vi "ble_read_hr_monitor.vi"() -> ()   [LabVIEW 2013]
uses:
  type_def/connection_status_bundle.ctl
  type_def/address_type.ctl
panel:
  out "Reading HR":bool
  in  "stop":bool
  out "HR (bpm)":u16
  out "Connected":bool
  out "Device Name":string
  in  "Address Type":T1=1 items=["Public", "Random"]
  out "Handle table":string[][](array[string])
  out "Connection Status":T2={"MAC Address"="", "cnx handle"=0, "cnx flags"=0, "Address Type"=125, "Connection Interval (ms)"=125, "Timeout(ms)"=125, "Latency"=0, "bonding handle"=0} {"Address Type" items=["Public", "Random"]}
  out "Scanning":bool
  in  "Continue":bool
  in  "MAC Address":string
  in  "COM Bluegiga in":refnum<visa-resource-name>="COM13"
  out "Devices":string[][](array[string])
  out "BLED112 Dongle Info":string
  # "This VI an example of scanning for BLE devices using the \nBLED112 Bluetooth Smart Dongle by Bluegiga\nhttps://www.bluegiga.com/en-US/products/bled112-bluetooth-smart-dongle/\nand\nBLE  toolkit for LabVIEW\n\nInstructions:\nBefore running the VI\n1. Select the COM port for the BLED112 USB receiver\n(You can verify this in the Device Manager)\n\n2. Run the VI\n\n3. The VI will reset the dongle and scan for available BLE devices\n \n4. Introduce the MAC Address and Address Type of the HR monitor to connect and click in the CONTINUE button to connect with it\n\nYour device MUST compy with the BLE Heart Rate Profile\nhttps://developer.bluetooth.org/TechnologyOverview/Pages/HRP.aspx\n\n5. The VI will read the Characteristic 0x2A00 of the Service 0x1800 which contains \nthe Device Name\n\nhttps://www.bluetooth.com/specifications/gatt/viewer?attributeXmlFile=org.bluetooth.service.generic_access.xml&u=org.bluetooth.service.generic_access.xml\n\n6. Hear rate value will be updated\n\n7. Click in STOP to end the Hear Rate acqusition"
  # "SCAN"
  # "RSSI (power)"
  # "Advertising Package Type"
  # "MAC Address"
  # "Address Type"
  # "Friendly name"
  # "DEVICES FOUND"
  # "Introduce the MAC Address and Address Type of the device you want to connect and click in the CONTINUE button"
  # "CONNECT"
  # "READING DATA FROM DEVICE"
  # "Service 0x1800\nCharacteristic 0x2A00\nDevice Name"
  # "Service 0x180D\nCharacteristic 0x2A37\nHeart Rate Measurement"
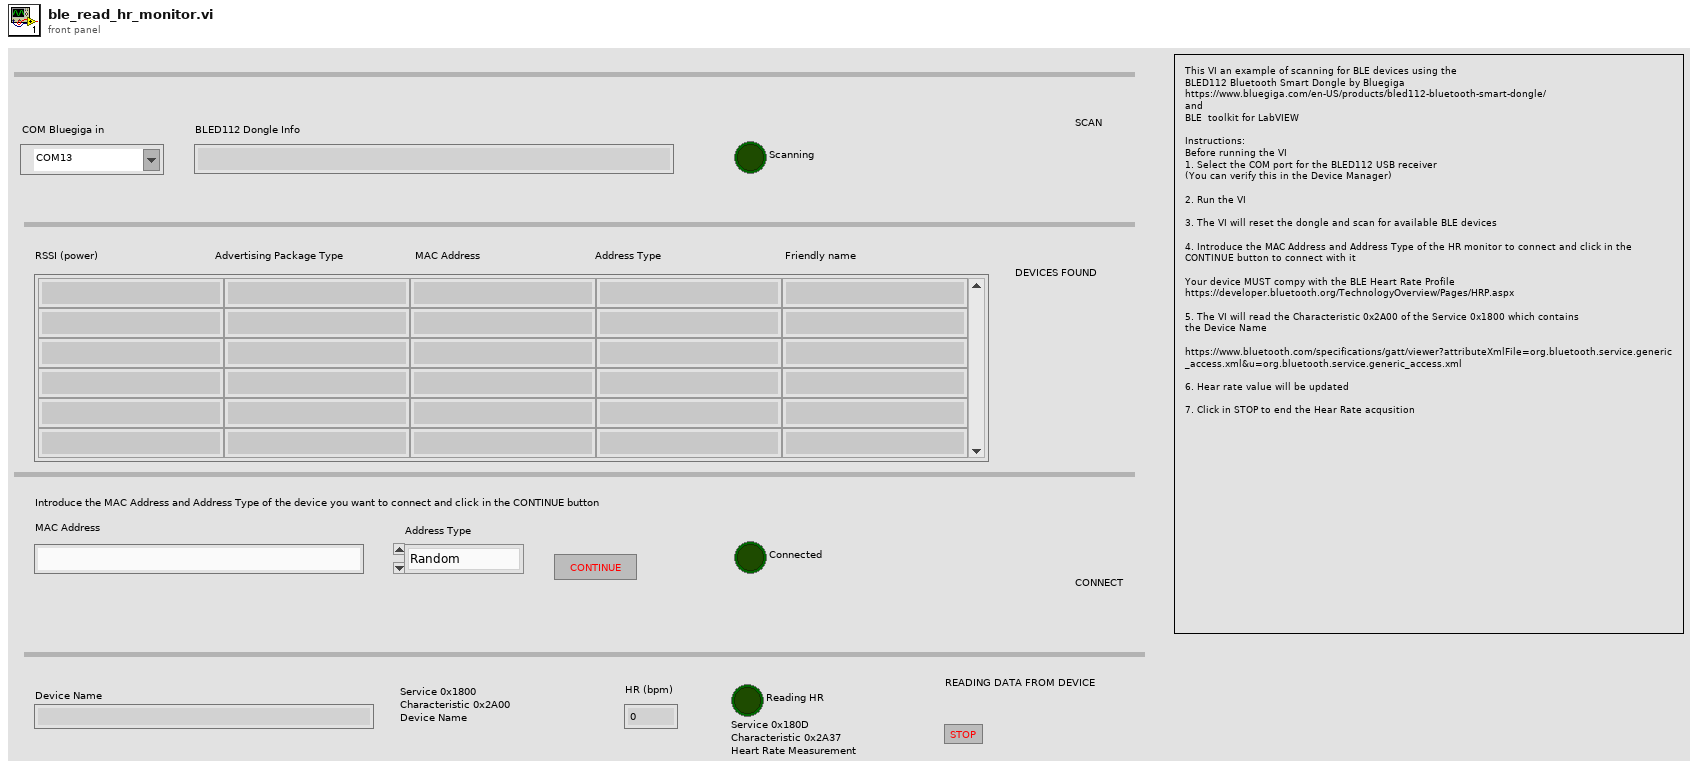
[diagram p1: front panel]
types:
  T1 = typedef "address_type.ctl" = u8
  T2 = typedef "connection_status_bundle.ctl" = cluster{"MAC Address":string, "cnx handle":u8, "cnx flags":u8, "Address Type":T1, "Connection Interval (ms)":u16, "Timeout(ms)":u16, "Latency":u16, "bonding handle":u8}
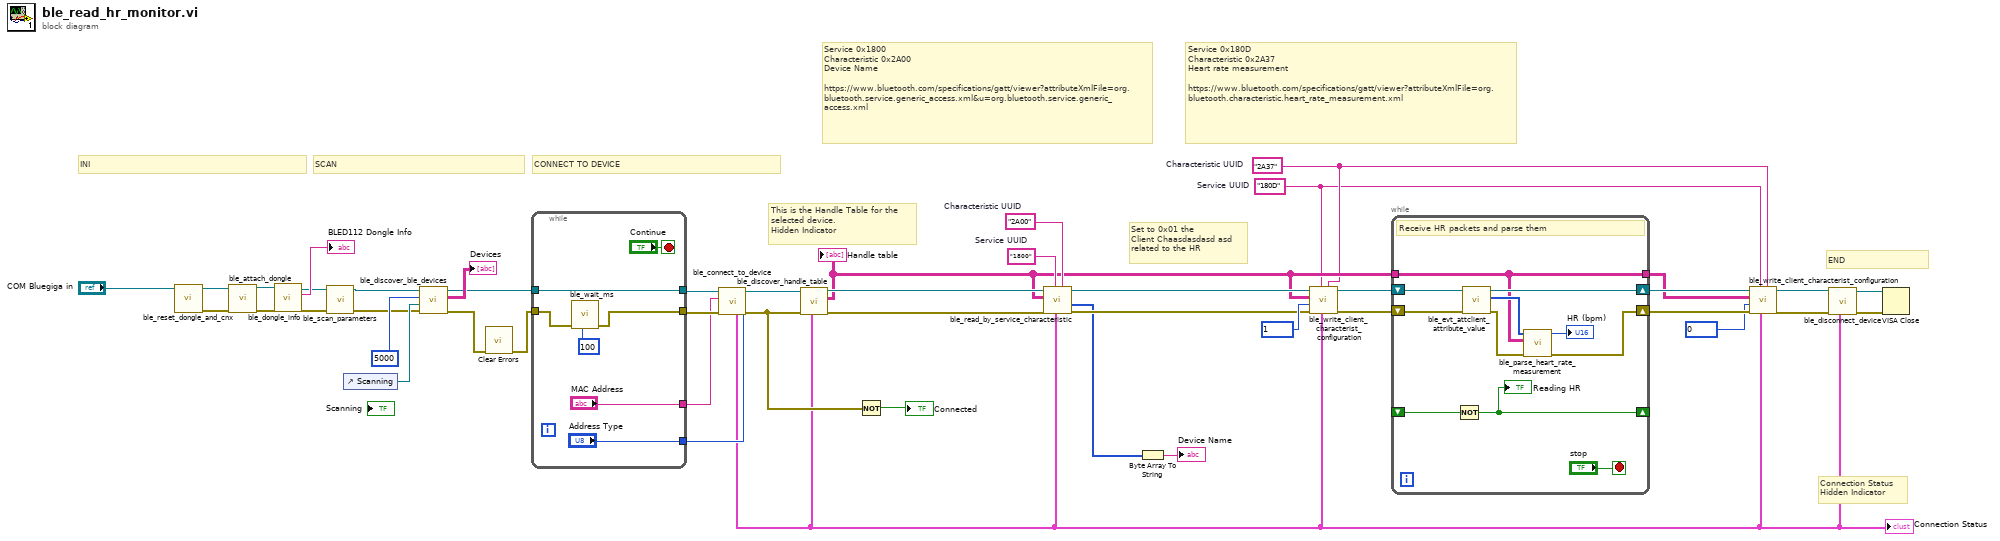
[diagram p0: block diagram]
diagram:
  w3 = "2A37"  # Characteristic UUID
  w2 = "180D"  # Service UUID
  w20 = "2A00"  # Characteristic UUID
  w21 = "1800"  # Service UUID
  # "Service 0x180D\nCharacteristic 0x2A37\nHeart rate measurement\n\nhttps://www.bluetooth.com/specifications/gatt/viewer?attributeXmlFile=org.bluetooth.characteristic.heart_rate_measurement.xml"
  # "Set to 0x01 the \nClient Chaasdasdasd asd\nrelated to the HR"
  # "Connection Status\nHidden Indicator"
  # "Service 0x1800\nCharacteristic 0x2A00\nDevice Name\n\nhttps://www.bluetooth.com/specifications/gatt/viewer?attributeXmlFile=org.bluetooth.service.generic_access.xml&u=org.bluetooth.service.generic_access.xml"
  # "This is the Handle Table for the\nselected device. \nHidden Indicator"
  # "CONNECT TO DEVICE"
  # "SCAN"
  # "END"
  # "INI"
  n1 = call "ble_reset_dongle_and_cnx.vi"("COM Bluegiga in"="COM Bluegiga in") -> ("error out"=w30:errorcluster, "COM Bluegiga out"=w28:refnum<visa-resource-name>)  [unwired: 9 in]
  n2 = call "ble_attach_dongle.vi"("error in (no error)"=w30, "COM Bluegiga in"=w28) -> ("error out"=w32:errorcluster, "COM Bluegiga out"=w31:refnum<visa-resource-name>)  [unwired: 8 in]
  n3 = call "ble_dongle_info.vi"("error in (no error)"=w32, "COM Bluegiga in"=w31) -> ("error out"=w38:errorcluster, "info"=→"BLED112 Dongle Info":string, "COM Bluegiga out"=w39:refnum<visa-resource-name>)  [unwired: 7 in]
  n4 = call "ble_scan_parameters.vi"("error in (no error)"=w38, "COM Bluegiga in"=w39) -> ("error out"=w36:errorcluster, "COM Bluegiga out"=w37:refnum<visa-resource-name>)  [unwired: 7 in, 1 out]
  n5 = control-ref of="Scanning"() -> (w42:refnum<vi>)
  n6 = call "ble_discover_ble_devices.vi"("error in (no error)"=w36, "LED ref"=w42, "Scan Duration (10000ms)"=u32 5000, "COM Bluegiga in"=w37) -> ("error out"=w26:errorcluster, "Devices"=→"Devices":string[][], "COM Bluegiga out"=w43:refnum<visa-resource-name>)  [unwired: 5 in]
  n7 = call <vilib>:"Clear Errors.vi"("error in (no error)"=w26) -> ("error out"=w25:errorcluster)  [unwired: 6 in]
  n8 = while {
    tunnel: w25 -> [w52]
    tunnel: [w51] -> w41
    tunnel: w43 -> [w51]
    tunnel: [w50] -> w40
    tunnel: ["MAC Address"] -> w33
    tunnel: ["Address Type"] -> w24
    stop <- "Continue" stop-if-true
    n9 = call "ble_wait_ms.vi"("milliseconds to wait (100)"=u32 100, "error in (no error)"=w52) -> ("error out"=w50:errorcluster)  [unwired: 9 in]
  }
  n10 = call "ble_connect_to_device.vi"("Address Type"=w24, "error in (no error)"=w40, "MAC Address"=w33, "COM Bluegiga in"=w41) -> ("error out"=w17:errorcluster, "COM Bluegiga out"=w27:refnum<visa-resource-name>, "Connection Status"=w9:T2)  [unwired: 5 in]
  "Connection Status" <- w9
  n11 = call "ble_discover_handle_table.vi"("Connection Status"=w9, "error in (no error)"=w17, "COM Bluegiga in"=w27) -> ("error out"=w23:errorcluster, "Handle table"=w4:string[][], "COM Bluegiga out"=w22:refnum<visa-resource-name>)  [unwired: 6 in]
  "Handle table" <- w4
  n12 = Not(x=w17) -> (.not. x?=→"Connected":bool)
  n13 = call "ble_read_by_service_characteristic.vi"("Characteristic UUID"=w20, "Connection Status"=w9, "Service UUID"=w21, "error in (no error)"=w23, "Handle table"=w4, "COM Bluegiga in"=w22) -> ("error out"=w6:errorcluster, "attribute value"=w1:u8[], "COM Bluegiga out"=w5:refnum<visa-resource-name>)  [unwired: 2 in, 1 out]
  n14 = Byte Array To String(unsigned byte array=w1) -> (string=→"Device Name":string)
  n15 = call "ble_write_client_characterist_configuration.vi"("Characteristic UUID"=w3, "Connection Status"=w9, "Service UUID"=w2, "error in (no error)"=w6, "Value(16bit)"=u16 1, "Handle table"=w4, "COM Bluegiga in"=w5) -> ("error out"=w16:errorcluster, "COM Bluegiga out"=w15:refnum<visa-resource-name>)  [unwired: 3 in]
  n16 = while {
    tunnel: w4 -> [w56]
    shift-right: [w58] -> w13
    shift-left: w15 -> [w62]
    shift-right: [w57] -> w14
    shift-left: w16 -> [w59]
    tunnel: [w56] -> w12
    shift-right: [w55] -> _
    shift-left: _ -> [w54]
    stop <- "stop" stop-if-true
    # "Receive HR packets and parse them"
    n17 = Not(x=w54) -> (.not. x?=w55:bool)
    "Reading HR" <- w55
    n18 = call "ble_evt_attclient_attribute_value.vi"("error in (no error)"=w59, "COM Bluegiga in"=w62) -> ("error out"=w63:errorcluster, "payload"=w64:u8[], "COM Bluegiga out"=w58:refnum<visa-resource-name>)  [unwired: 5 in, 2 out]
    n19 = call "ble_parse_heart_rate_measurement.vi"("error in (no error)"=w63, "Handle table"=w56, "payload"=w64) -> ("error out"=w57:errorcluster, "HR (bpm)"=→"HR (bpm)":u16)  [unwired: 6 in, 1 out]
  }
  n20 = call "ble_write_client_characterist_configuration.vi"("Characteristic UUID"=w3, "Connection Status"=w9, "Service UUID"=w2, "error in (no error)"=w14, "Value(16bit)"=u16 0, "Handle table"=w12, "COM Bluegiga in"=w13) -> ("error out"=w10:errorcluster, "COM Bluegiga out"=w11:refnum<visa-resource-name>)  [unwired: 3 in]
  n21 = call "ble_disconnect_device.vi"("Connection Status"=w9, "error in (no error)"=w10, "COM Bluegiga in"=w11) -> ("error out"=w34:errorcluster, "COM Bluegiga out"=w35:refnum<visa-resource-name>)  [unwired: 7 in]
  n22 = VISA Close(VISA resource name=w35, error in (no error)=w34) -> ()  [unwired: 1 out]
